vi "Exsample Grid Main.vi"() -> ()   [LabVIEW 2016]
uses:
  Grid Parameter.ctl
panel:
  in  "表":string[][](table)
  # "範囲チェックは、別途作成したクラスタ\n（Exsample Grid Cluster.vi）を考慮して\n自動丸めを実施。"
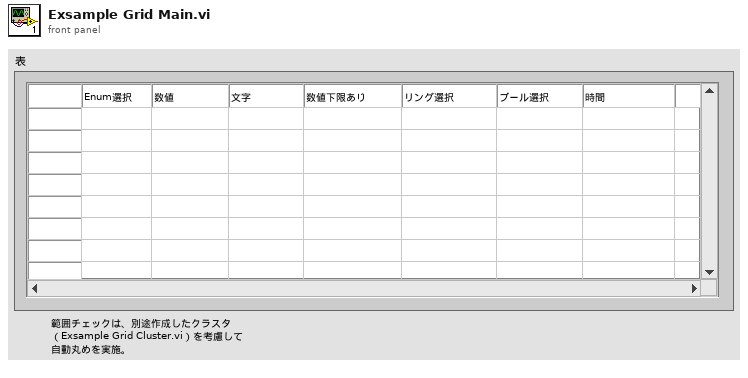
[diagram p1: front panel]
types:
  T1 = typedef "Grid Parameter.ctl" = cluster{"ref.制御器[]":refnum<vi>[], "ref.表":refnum<vi>, "表サイズ(縦×横)":i32[]}
  T2 = typedef "eventvkey.ctl" = enum16{"ASCII", "Enter", "Return", "Shift", "Ctrl", "Alt", "Cmd", "Opt", "Caps", "NumLock", "Clear", "Break", "Up", "Down", "Left", "Right", "Insert", "Delete", "Home", "End", "PageUp", "PageDown", "Escape", "Help", "Pause", "ScrollLock", "F1", "F2", "F3", "F4", "F5", "F6", "F7", "F8", "F9", "F10", "F11", "F12", "F13", "F14", "F15", "F16", "F17", "F18", "F19", "F20", "F21", "F22", "F23", "F24", "Play", "VolumeUp", "VolumeDown", "Mute", "Two Byte Char"}
  T3 = cluster{"Shift":bool, "Ctrl":bool, "Alt":bool, "Cmd":bool, "Opt":bool}
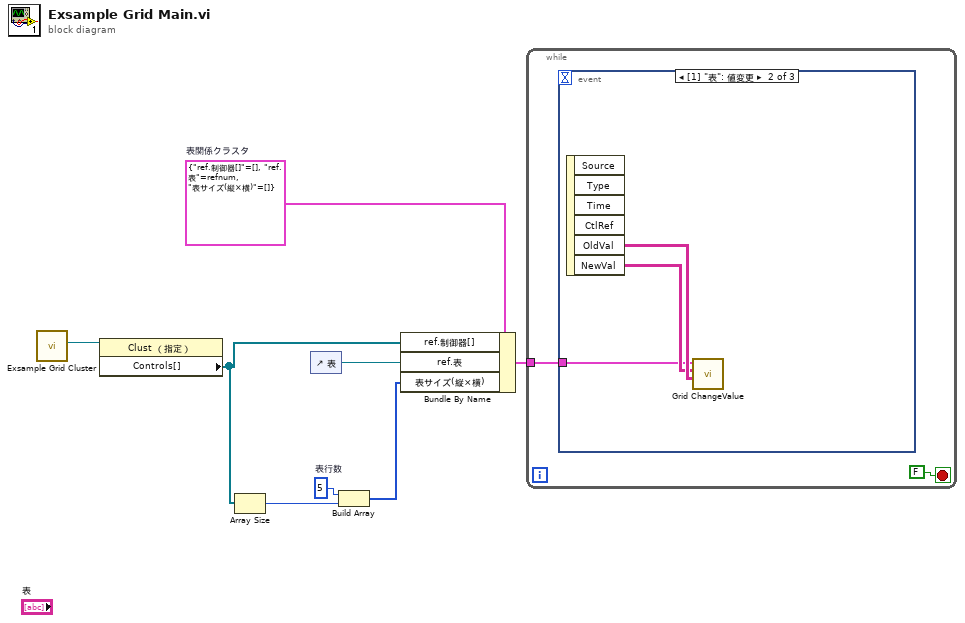
[diagram p0: block diagram]
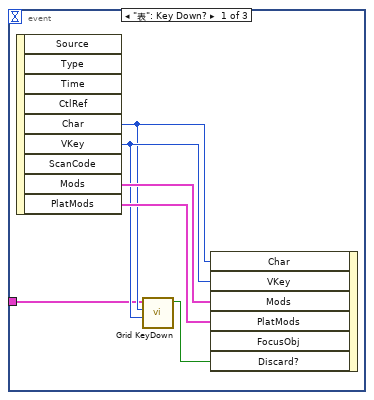
[diagram p2: hidden frame]
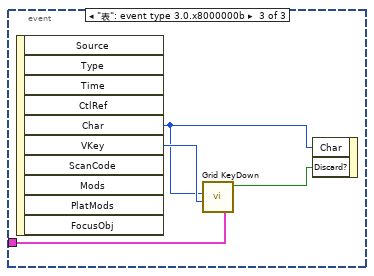
[diagram p3: hidden frame]
diagram:
  w3 = T1 {"ref.制御器[]"=[], "ref.表"=refnum, "表サイズ(縦×横)"=[]}  # 表関係クラスタ
  w7 = 5  # 表行数
  n1 = call "Exsample Grid Cluster.vi"() -> ("ref.条件クラスタ"=w2:refnum<vi>)  [unwired: 11 in]
  n2 = property class="Clust （指定）"(reference=w2) -> ("Controls[]"=w1:refnum<vi>[])  [unwired: 1 in, 2 out]
  n3 = Array Size(array=w1) -> (size(s)=w8:i32)
  n4 = control-ref of="表"() -> (w6:refnum<vi>)
  n5 = Build Array(w7, w8) -> (w5:i32[])
  n6 = Bundle By Name(cluster=w3, "ref.制御器[]"=w1, "ref.表"=w6, "表サイズ(縦×横)"=w5) -> (w4:T1)
  n7 = while {
    tunnel: w4 -> [w9]
    stop <- FALSE stop-if-true
    n8 = event shown="[1] \"表\": 値変更" {
      selector: _ -> [_ _ _]
      dyn-events: _ -> [_ _ _]
      timeout: _ -> [_ _ _]
      tunnel: w9 -> [w11 w17 w23]
      event "表": Key Down? {
        n9 = event-data() -> ("Char"=w12:i16, "VKey"=w13:T2, "Mods"=w14:cluster{"Num Pad":bool, "Menu Key":bool}, "PlatMods"=w15:T3)  [unwired: 1 in, 5 out]
        n10 = call "Grid KeyDown.vi"("VKey"=w13, "Char"=w12, "表関係クラスタ"=w11) -> ("破棄?"=w16:bool)  [unwired: 7 in, 1 out]
        n11 = event-data("Char"=w12, "VKey"=w13, "Mods"=w14, "PlatMods"=w15, "Discard?"=w16) -> ()  [unwired: 2 in, 1 out]
      }
      event "表": Value Change {
        n12 = event-data() -> ("OldVal"=w19:string[][], "NewVal"=w18:string[][])  [unwired: 1 in, 4 out]
        n13 = call "Grid ChangeValue.vi"("OldVal"=w19, "NewVal"=w18, "出力クラスタ"=w17) -> ()  [unwired: 6 in, 3 out]
      }
      event "表": event type 3.0.x8000000b {
        n14 = event-data() -> ("Char"=w20:i16, "VKey"=w22:T2)  [unwired: 1 in, 8 out]
        n15 = call "Grid KeyDown.vi"("VKey"=w22, "Char"=w20, "表関係クラスタ"=w23) -> ("破棄?"=w21:bool)  [unwired: 7 in, 1 out]
        n16 = event-data("Char"=w20, "Discard?"=w21) -> ()  [unwired: 1 in, 1 out]
      }
    }
  }
